vi "GET_issue_lastupdates_by_ids.vi"(8 "error in (no error)":errorcluster, 9 "offset":i32, 10 "volume id":i32, 11 "REST Client in":refnum<class "REST Client.lvclass">) -> (0 "error out":errorcluster, 2 "results":T1, 3 "REST Client out":refnum<class "REST Client.lvclass">)   [LabVIEW 2024, in "CV_RESTful_Lib.lvlib"]
uses:
  CV_RESTful_Lib.lvlib
  <vilib>/addons/_JKI.lib/REST Client/classes/REST Client/REST Client.lvclass
  typedefs/cv_date_updated.results--array.ctl
  <vilib>/addons/_JKI.lib/REST Client/classes/REST Client/HTTP Header.ctl
  <vilib>/NI/Advanced HTTP Client/Header--Combo Box.ctl
  typedefs/cv_date_updated--cluster.ctl
  <vilib>/NI/Advanced HTTP Client/Session.lvclass
  <vilib>/addons/_JKI.lib/Serialization/JSON/JKI JSON Serialization.lvlib
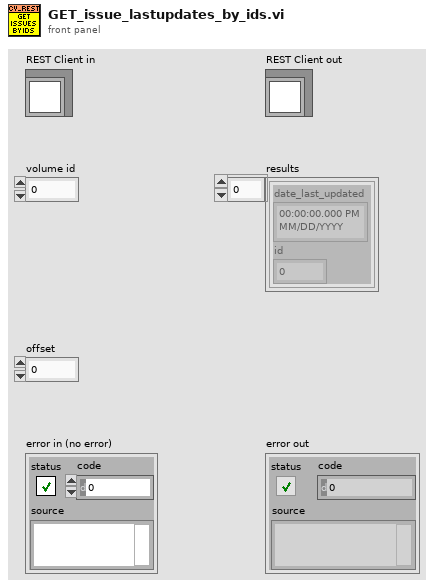
[diagram p1: front panel]
types:
  T1 = typedef "CV_RESTful_Lib.lvlib/cv_date_updated.results--array.ctl" = cluster{"date_last_updated":timestamp, "id":i32}[]
  T2 = typedef "CV_RESTful_Lib.lvlib/cv_date_updated--cluster.ctl" = cluster{"status_code":i32, "number_of_total_results":i32, "number_of_page_results":i32, "offset":i32, "limit":i32, "error":string, "results":T1}
  T3 = typedef "REST Client.lvlib/REST Client.lvclass/HTTP Header.ctl" = cluster{"header":T4, "value":string}
  T4 = typedef "lib_NI_Advanced HTTP Client.lvlib/Session.lvclass/Header--Combo Box.ctl" = string
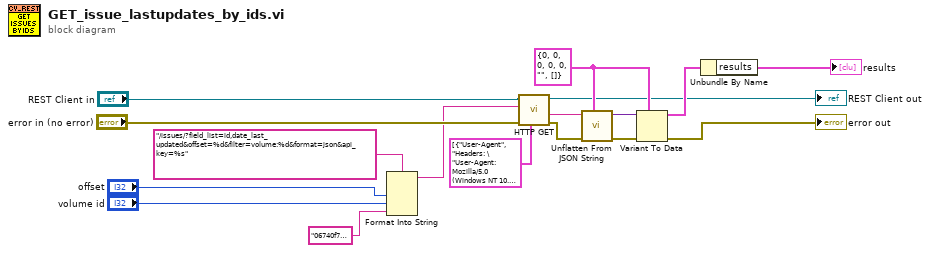
[diagram p0: block diagram]
diagram:
  w9 = T2 {"status_code"=0, "number_of_total_results"=0, "number_of_page_results"=0, "offset"=0, "limit"=0, "error"="", "results"=[]} ("Last Updated")
  n1 = Format Into String(format string="/issues/?field_list=id,date_last_updated&offset=%d&filter=volume:%d&format=json&api_key=%s", "offset", "volume id", "06740f73403e0b211d597c50ea94c7f16ea5e8ea") -> (resulting string=w12:string)  [unwired: 2 in, 1 out]
  n2 = call-dynamic "HTTP GET.vi"("request specific headers"=T3[] [{"header"="User-Agent", "value"="Headers: \"User-Agent: Mozilla/5.0 (Windows NT 10.0; Win64; x64) AppleWebKit/537.36 (KHTML, like Gecko) Chrome/91.0.4472.101 Safari/537.36\""}], "error in (no error)"="error in (no error)", "Path"=w12, "REST Client in"="REST Client in") -> ("error out"=w17:errorcluster, "Response body"=w13:string, "REST Client out"=→"REST Client out":refnum<class "REST Client.lvclass">)  [unwired: 2 in, 3 out]
  n3 = call <vilib>:"Unflatten From JSON String.vi"("Type and Defaults"=w9, "error in"=w17, "JSON String"=w13) -> ("error out"=w11:errorcluster, "Variant"=w10:variant)  [unwired: 7 in]
  n4 = Variant To Data(error in=w11, type=w9, Variant=w10) -> (data=w8:T2, error out=→"error out":errorcluster)
  n5 = Unbundle By Name(w8) -> ("results"=→"results":T1)
